vi "Read Trigger_TargetsRef.vi"(8 "error in (no error)":errorcluster, 11 "Electronic Load in":refnum<class "Electronic Load.lvclass">) -> (0 "error out":errorcluster, 2 "Trigger_TargetsRef":refnum<vi>, 3 "Electronic Load out":refnum<class "Electronic Load.lvclass">)   [LabVIEW 2019, in "Electronic Load.lvlib" / "Electronic Load.lvclass"]
uses:
  Library/Electronic Load.lvclass
  Library/Electronic Load.lvclass/Electronic Load.ctl
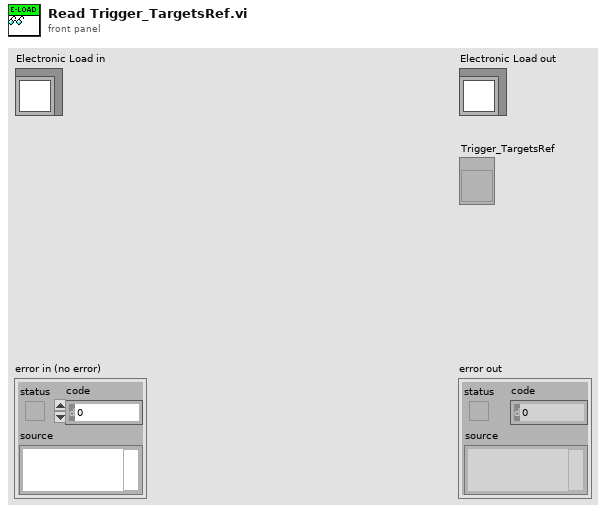
[diagram p1: front panel]
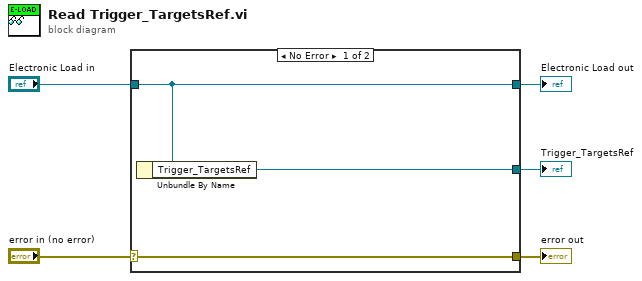
[diagram p0: block diagram]
diagram:
  n1 = case shown="No Error" "error in (no error)" {
    selector: "error in (no error)" -> [w8 w9]
    tunnel: [w8 w9] -> w4
    tunnel: [w7 w10] -> w2
    tunnel: "Electronic Load in" -> [w7 w10]
    tunnel: [w6 _] -> w1
    frame No Error {
      n2 = Unbundle By Name(w7) -> ("Trigger_TargetsRef"=w6:refnum<vi>)
    }
    frame Error {
    }
  }
  "error out" <- w4
  "Electronic Load out" <- w2
  "Trigger_TargetsRef" <- w1
